vi "Send Configure Output Mode.vi"(7 "Message Priority (Normal)":T1=enum."Normal", 8 "error in (no error)":errorcluster, 10 "output mode (Standard Function)":i32(ring) items=["Standard Function", "Arbitrary Waveform", "Arbitrary Sequence"], 11 "Message Enqueuer":refnum<class "Message Enqueuer.lvclass">) -> (0 "error out":errorcluster, 3 "Message Enqueuer out":refnum<class "Message Enqueuer.lvclass">)   [LabVIEW 2015, in "CS++Fgen.lvlib" / "Configure Output Mode Msg.lvclass"]
doc: "Sends the <B>CS++Fgen.lvlib:Configure Output Mode Msg.lvclass</B> message.\n\n<B>CS++Fgen.lvlib:CS++Fgen.lvclass:Configure Output Mode.vi</B> Description:\n\nThis VI configures the output mode of the function generator. The output mode determines the kind of waveform the function generator produces. For example, you can select to output a standard waveform, an arbitrary waveform, or a sequence of arbitrary waveforms."
uses:
  Configure Output Mode Msg.lvclass
  <vilib>/ActorFramework/Message Enqueuer/Message Enqueuer.lvclass
  <vilib>/ActorFramework/Message Enqueuer/Message Priority.ctl
  Configure Output Mode Msg.lvclass/Configure Output Mode Msg.ctl
  <vilib>/ActorFramework/Message Enqueuer/Message Enqueuer.lvclass/Message Enqueuer.ctl
  <vilib>/ActorFramework/Message Priority Queue/Priority Enqueue.vi
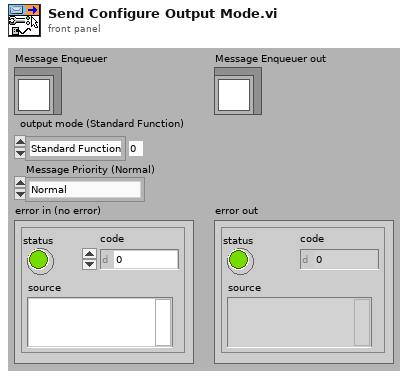
[diagram p1: front panel]
types:
  T1 = typedef "Actor Framework.lvlib/Message Enqueuer.lvclass/Message Priority.ctl" = enum16{"Low", "Normal", "High"}
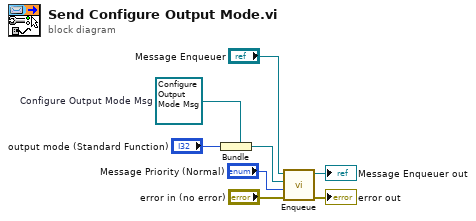
[diagram p0: block diagram]
diagram:
  w2 = refnum<class "Configure Output Mode Msg.lvclass"> refnum  # Configure Output Mode Msg
  n1 = Bundle(cluster=w2, "output mode (Standard Function)") -> (w5:refnum<class "Configure Output Mode Msg.lvclass">)
  n2 = call <vilib>:"Enqueue.vi"("error in (no error)"="error in (no error)", "Message Priority (Normal)"="Message Priority (Normal)", "Message"=w5, "Message Enqueuer in"="Message Enqueuer") -> ("error out"=→"error out":errorcluster, "Message Enqueuer out"=→"Message Enqueuer out":refnum<class "Message Enqueuer.lvclass">)  [unwired: 6 in]
